vi "Write isRoot.vi"(8 "error in (no error)":errorcluster, 10 "isRoot":bool, 11 "Engine in":refnum<class "Engine.lvclass">) -> (0 "error out":errorcluster, 3 "Engine out":refnum<class "Engine.lvclass">)   [LabVIEW 2019, in "Engine.lvlib" / "Engine.lvclass"]
uses:
  Project/Engine.lvclass
  Project/Engine.lvclass/Engine.ctl
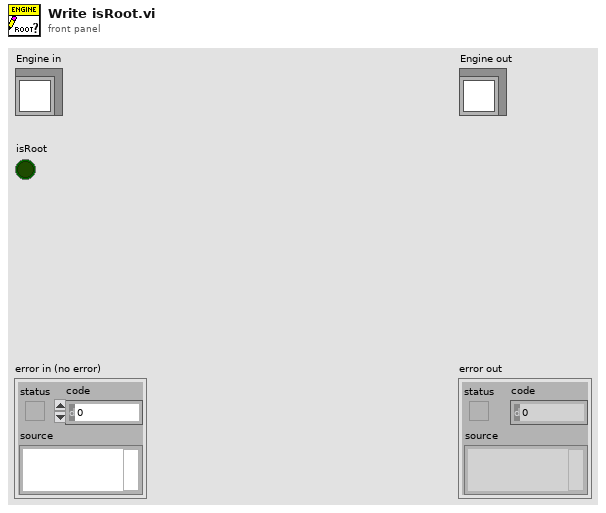
[diagram p1: front panel]
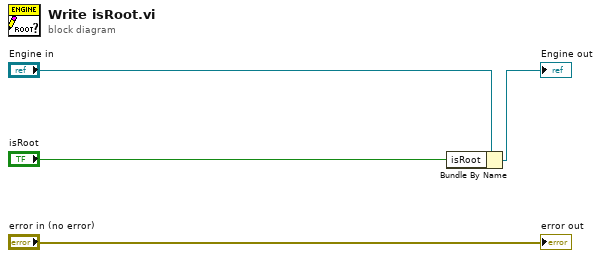
[diagram p0: block diagram]
diagram:
  n1 = Bundle By Name(cluster="Engine in", "isRoot"="isRoot") -> (→"Engine out":refnum<class "Engine.lvclass">)
  "error out" <- "error in (no error)"
